vi "Get FPGA Settings.vi"(8 "error in (no error)":errorcluster, 11 "Item Ref in":T2 format="%.0x") -> (0 "error out":errorcluster, 2 "FPGA Bitfile Settings":T1, 3 "Item Ref out":T2=18446744073709551615 format="%.0x")   [LabVIEW 2015, in "J1939 Addon System Explorer.lvlib"]
uses:
  J1939 Addon System Explorer.lvlib
  <vilib>/NI Veristand/Custom Device API/Custom Device Item Ref.ctl
  Shared/Types/SysDef FPGA Settings.ctl
  <vilib>/NI Veristand/Custom Device API/Get Item Property (Path).vi
  <vilib>/NI Veristand/Custom Device API/Get Item Property (U16).vi
  Shared/SubVIs/Constants.vi
  <vilib>/NI Veristand/Custom Device API/Get Item Property (Boolean).vi
  <vilib>/NI VeriStand/Custom Device API/Custom Device API.lvlib
  Shared/J1939 Addon Shared.lvlib
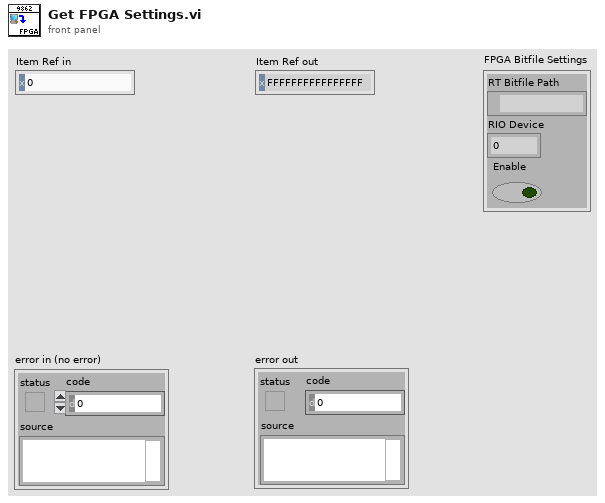
[diagram p1: front panel]
types:
  T1 = typedef "J1939 Addon Shared.lvlib/SysDef FPGA Settings.ctl" = cluster{"RT Bitfile Path":path, "RIO Device":u16, "Enable":bool}
  T2 = typedef "Custom Device API.lvlib/Custom Device Item Ref.ctl" = u64
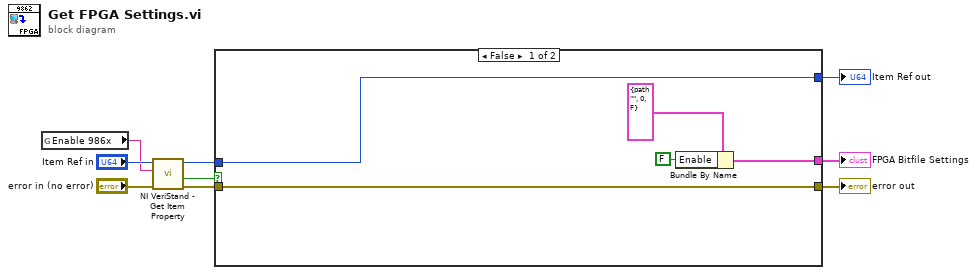
[diagram p0: block diagram]
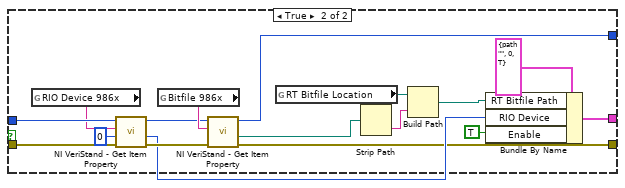
[diagram p2: hidden frame]
diagram:
  n1 = global read "Constants.vi" "Enable 986x"() -> (w4:string)
  n2 = call-poly <vilib>:"NI VeriStand - Get Item Property.vi"("error in (no error)"="error in (no error)", "Property Name"=w4, "Item Ref in"="Item Ref in") -> ("error out"=w2:errorcluster, "Value"=w3:bool, "Item Ref out"=w9:T2)  [unwired: 5 in, 1 out]
  n3 = case shown="False" w3 {
    tunnel: w9 -> [w13 w27]
    tunnel: w2 -> [w14 w29]
    tunnel: [w14 w17] -> w8
    tunnel: [w13 w31] -> w5
    tunnel: [w11 w16] -> w1
    frame False {
      n4 = Bundle By Name(cluster=T1 {"RT Bitfile Path"=path "", "RIO Device"=0, "Enable"=FALSE}, "Enable"=FALSE) -> (w11:T1)
    }
    frame True {
      n5 = global read "Constants.vi" "RIO Device 986x"() -> (w25:string)
      n6 = call-poly <vilib>:"NI VeriStand - Get Item Property.vi"("error in (no error)"=w29, "Default Value"=u16 0, "Property Name"=w25, "Item Ref in"=w27) -> ("error out"=w28:errorcluster, "Value"=w18:u16, "Item Ref out"=w26:T2)  [unwired: 4 in, 1 out]
      n7 = global read "Constants.vi" "Bitfile 986x"() -> (w30:string)
      n8 = call-poly <vilib>:"NI VeriStand - Get Item Property.vi"("error in (no error)"=w28, "Property Name"=w30, "Item Ref in"=w26) -> ("error out"=w17:errorcluster, "Value"=w21:path, "Item Ref out"=w31:T2)  [unwired: 5 in, 1 out]
      n9 = global read "Constants.vi" "RT Bitfile Location"() -> (w22:path)
      n10 = Strip Path(path=w21) -> (name=w23:string)  [unwired: 1 out]
      n11 = Build Path(base path=w22, name or relative path=w23) -> (appended path=w19:path)
      n12 = Bundle By Name(cluster=T1 {"RT Bitfile Path"=path "", "RIO Device"=0, "Enable"=TRUE}, "RT Bitfile Path"=w19, "RIO Device"=w18, "Enable"=TRUE) -> (w16:T1)
    }
  }
  "error out" <- w8
  "Item Ref out" <- w5
  "FPGA Bitfile Settings" <- w1
